vi "Update Slot Configuration.vi"(6 "Max # of Racks":u16, 8 "error in (no error)":errorcluster, 9 "Card Position":T1[](array[typedef]) {"Slot #" max=15}, 10 "Card Name":string[](array[string]), 11 "Slot Configuration in":refnum<vi>) -> (0 "error out":errorcluster, 3 "Slot Configuration out":refnum<vi>)   [LabVIEW 2014, in "SLSC configuration System Explorer.lvlib"]
uses:
  SLSC configuration System Explorer.lvlib
  Type Defs/Card Position.ctl
  Shared/SPI Utility/Slot #.ctl
  <vilib>/Utility/miscctls.llb/LVRowAndColumnTypeDef.ctl
  Shared/Constants.vi
  Shared/SLSC configuration Shared.lvlib
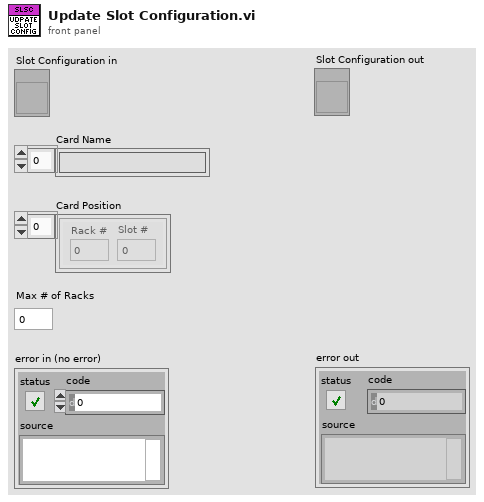
[diagram p1: front panel]
types:
  T1 = typedef "SLSC configuration Shared.lvlib/Card Position.ctl" = cluster{"Rack #":u8, "Slot #":T2}
  T2 = typedef "SLSC configuration Shared.lvlib/Slot #.ctl" = u8
  T3 = typedef "LVRowAndColumnTypeDef.ctl" = cluster{"Row":i32, "Column":i32}
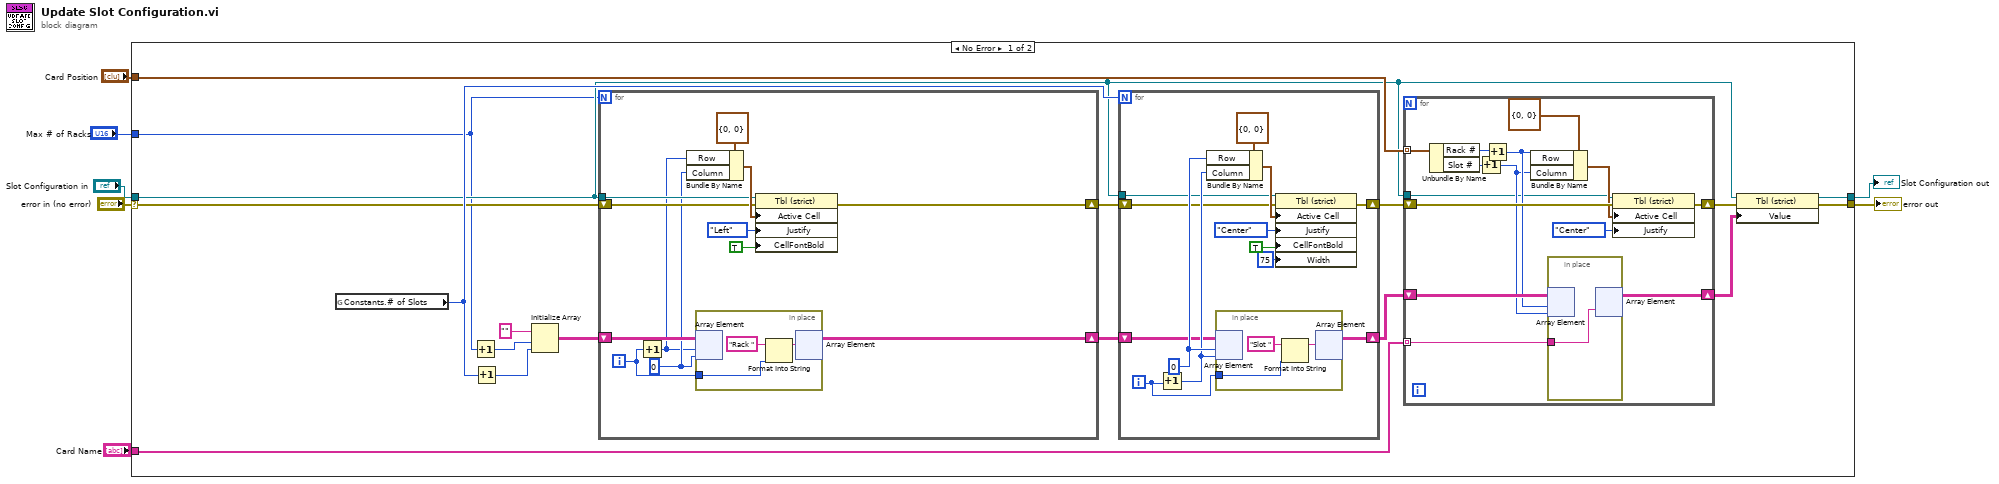
[diagram p0: block diagram]
diagram:
  n1 = case shown="No Error" "error in (no error)" {
    selector: "error in (no error)" -> [w14 w72]
    tunnel: "Card Position" -> [w23 _]
    tunnel: "Card Name" -> [w22 _]
    tunnel: [w12 w72] -> w2
    tunnel: "Slot Configuration in" -> [w9 w73]
    tunnel: [w10 w73] -> w3
    tunnel: "Max # of Racks" -> [w8 _]
    frame No Error {
      n2 = global read "Constants.vi" "Constants.# of Slots"() -> (w15:u8)
      n3 = Increment(x=w8) -> (x+1=w24:u16)
      n4 = Increment(x=w15) -> (x+1=w16:u8)
      n5 = Initialize Array("", w24, w16) -> (w21:string[][])
      n6 = for {
        N: w8 -> [_]
        shift-right: [w42] -> w20
        shift-left: w21 -> [w53]
        shift-right: [w43] -> w19
        shift-left: w14 -> [w49]
        tunnel: w9 -> [w48]
        i -> [w45]
        w46 = 0
        n7 = Increment(x=w45) -> (x+1=w44:i32)
        n8 = Bundle By Name(cluster=T3 {"Row"=0, "Column"=0} ("Active Cell:Active Cell"), "Row"=w44, "Column"=w46) -> (w51:T3)
        n9 = in-place {
          in-place-border: w45 -> [w56]
          n10 = in-place-array #1(w53, w44, w46) -> ()  [unwired: 1 out]
          n11 = Format Into String(initial string="Rack ", w56) -> (resulting string=w54:string)  [unwired: 2 in, 1 out]
          n12 = in-place-array #1(w54) -> (w42:string[][])  [unwired: 2 out]
        }
        n13 = property class="Tbl (strict)"(reference=w48, error in=w49, "Active Cell"=w51, "Justify"=enum16{"Left", "Center", "Right"}."Left" ("Active Cell:Cell Justification"), "CellFontBold"=TRUE ("Active Cell:Cell Font:Bold")) -> (error out=w43:errorcluster)  [unwired: 1 out]
      }
      n14 = for {
        N: w15 -> [_]
        shift-right: [w28] -> w18
        shift-left: w20 -> [w29]
        shift-right: [w27] -> w17
        shift-left: w19 -> [w31]
        tunnel: w9 -> [w30]
        i -> [w34]
        w33 = 0
        n15 = Increment(x=w34) -> (x+1=w32:i32)
        n16 = Bundle By Name(cluster=T3 {"Row"=0, "Column"=0} ("Active Cell:Active Cell"), "Row"=w33, "Column"=w32) -> (w37:T3)
        n17 = in-place {
          in-place-border: w34 -> [w41]
          n18 = in-place-array #2(w29, w33, w32) -> ()  [unwired: 1 out]
          n19 = Format Into String(initial string="Slot ", w41) -> (resulting string=w39:string)  [unwired: 2 in, 1 out]
          n20 = in-place-array #2(w39) -> (w28:string[][])  [unwired: 2 out]
        }
        n21 = property class="Tbl (strict)"(reference=w30, error in=w31, "Active Cell"=w37, "Justify"=enum16{"Left", "Center", "Right"}."Center" ("Active Cell:Cell Justification"), "CellFontBold"=TRUE ("Active Cell:Cell Font:Bold"), "Width"=u32 75 ("Active Cell:Cell Size:Width")) -> (error out=w27:errorcluster)  [unwired: 1 out]
      }
      n22 = for {
        tunnel: w23 -> [w69] mode=indexing
        shift-right: [w62] -> w11
        shift-left: w18 -> [w64]
        tunnel: w22 -> [w63] mode=indexing
        shift-right: [w65] -> w13
        shift-left: w17 -> [w70]
        tunnel: w9 -> [w57]
        n23 = Unbundle By Name(w69) -> ("Rack #"=w60:u8, "Slot #"=w61:T2)
        n24 = Increment(x=w61) -> (x+1=w58:T2)
        n25 = Increment(x=w60) -> (x+1=w59:u8)
        n26 = Bundle By Name(cluster=T3 {"Row"=0, "Column"=0} ("Active Cell:Active Cell"), "Row"=w59, "Column"=w58) -> (w67:T3)
        n27 = in-place {
          in-place-border: w63 -> [w71]
          n28 = in-place-array #3(w64, w59, w58) -> ()  [unwired: 1 out]
          n29 = in-place-array #3(w71) -> (w62:string[][])  [unwired: 2 out]
        }
        n30 = property class="Tbl (strict)"(reference=w57, error in=w70, "Active Cell"=w67, "Justify"=enum16{"Left", "Center", "Right"}."Center" ("Active Cell:Cell Justification")) -> (error out=w65:errorcluster)  [unwired: 1 out]
      }
      n31 = property class="Tbl (strict)"(reference=w9, error in=w13, "Value"=w11) -> (reference out=w10:refnum<vi>, error out=w12:errorcluster)
    }
    frame Error {
    }
  }
  "error out" <- w2
  "Slot Configuration out" <- w3
